vi "fgv_3d_imu.vi"(7 "cmd":enum16{"ini", "update"}(ring), 11 "3d cfg":cluster{"x":dbl, "y":dbl, "z":dbl}={"x"=1.0, "y"=1.0, "z"=1.0}) -> ()   [LabVIEW 2019]
uses:
  <vilib>/picture/3D Picture Control/Object/Create Object (name).vi
  <vilib>/picture/3D Picture Control/NI_3D Picture Control.lvlib
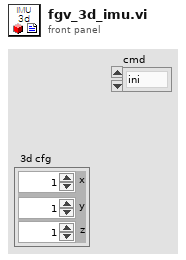
[diagram p1: front panel]
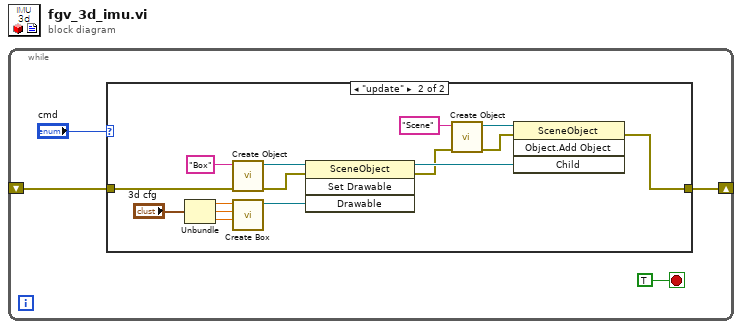
[diagram p0: block diagram]
diagram:
  n1 = while {
    shift-right: [w1] -> _
    shift-left: _ -> [w2]
    stop <- TRUE stop-if-true
    n2 = case shown="\"update\"" "cmd" {
      tunnel: w2 -> [w5 w11]
      tunnel: [w5 w10] -> w1
      frame "ini", Default {
      }
      frame "update" {
        n3 = Unbundle("3d cfg") -> ("x"=w8:dbl, "y"=w7:dbl, "z"=w6:dbl)
        n4 = call-poly <vilib>:"Create Object.vi"("error in (no error)"=w11, "Name"="Box") -> ("error out"=w15:errorcluster, "Scene:New Object"=w14:refnum<vi>)  [unwired: 8 in]
        n5 = call <vilib>:"Create Box.vi"("Length Z"=w6, "Length Y"=w7, "Length X"=w8) -> ("New Box Refnum"=w16:refnum<vi>)  [unwired: 7 in, 1 out]
        n6 = invoke class="SceneObject" method="Set Drawable"(reference=w14, error in=w15, "Drawable"=w16) -> (reference out=w20:refnum<vi>, error out=w12:errorcluster)  [unwired: 1 in, 2 out]
        n7 = call-poly <vilib>:"Create Object.vi"("error in (no error)"=w12, "Name"="Scene") -> ("error out"=w19:errorcluster, "Scene:New Object"=w18:refnum<vi>)  [unwired: 8 in]
        n8 = invoke class="SceneObject" method="Object.Add Object"(reference=w18, error in=w19, "Child"=w20) -> (error out=w10:errorcluster)  [unwired: 1 in, 3 out]
      }
    }
  }
